vi "Data file Conversion.vi"() -> ()   [LabVIEW 2020]
uses:
  <vilib>/Utility/sysdir.llb/System Directory Type.ctl
  <vilib>/Utility/NIReport.llb/Report Type.ctl
  <vilib>/addons/_office/excel.llb/Excel Get Data ([str]).vi
  <vilib>/Utility/file.llb/Write Delimited Spreadsheet (string).vi
  <vilib>/Utility/NIReport.llb/NI_report.lvclass
  <vilib>/addons/_office/NI_ReportGenerationToolkit.lvlib
  <vilib>/Utility/NIReport.llb/Excel/NI_Excel.lvclass
  <vilib>/Utility/NIReport.llb/NI_ReportGenerationCore.lvlib
panel:
  out "data 2":string[][][](array[string])
  out "data":string[][](array[string])
  out "error out":errorcluster caption="에러 출력"
  in  "파일선택":T1(ring)=enum."Torque Weight Set"
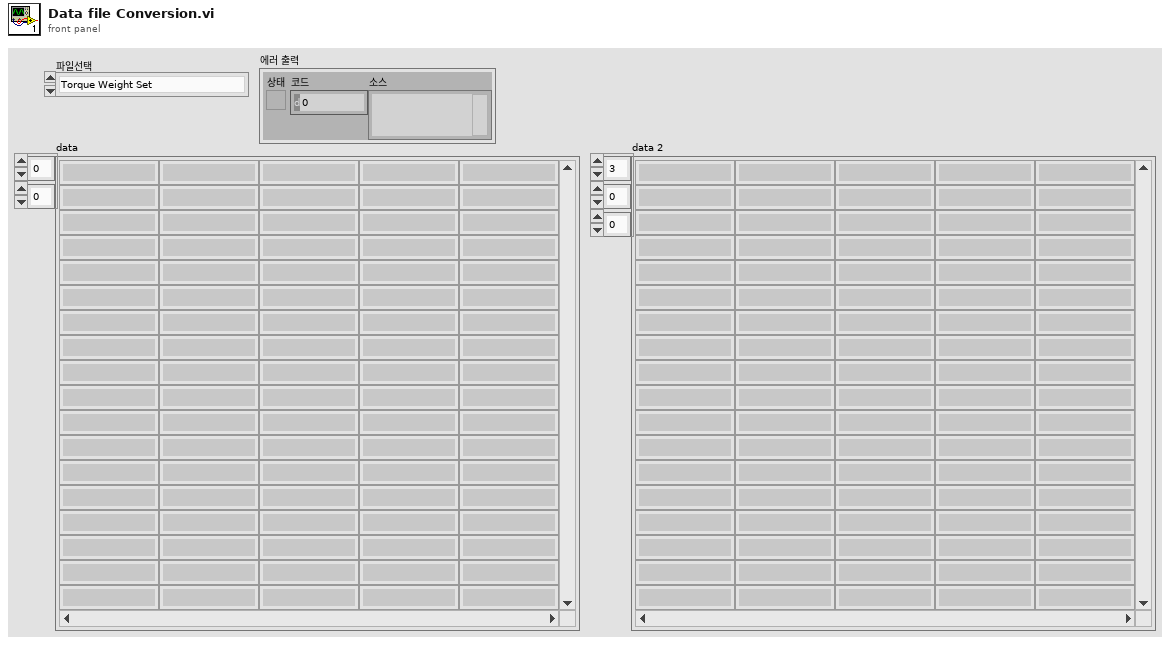
[diagram p1: front panel]
types:
  T1 = enum16{"Force Weight Set", "Torque Weight Set", "Deadweight Set", "Gauge Block Set", "Angle Gauge Block Set", "Thread Plug Gauge Set", "Surface Plate"}
  T2 = typedef "NI_ReportGenerationCore.lvlib/Report Type.ctl" = enum16{"HTML", "Word", "Excel"}
  T3 = enum16{"maximized", "minimized", "normal", "no change"}
  T4 = typedef "System Directory Type.ctl" = i32
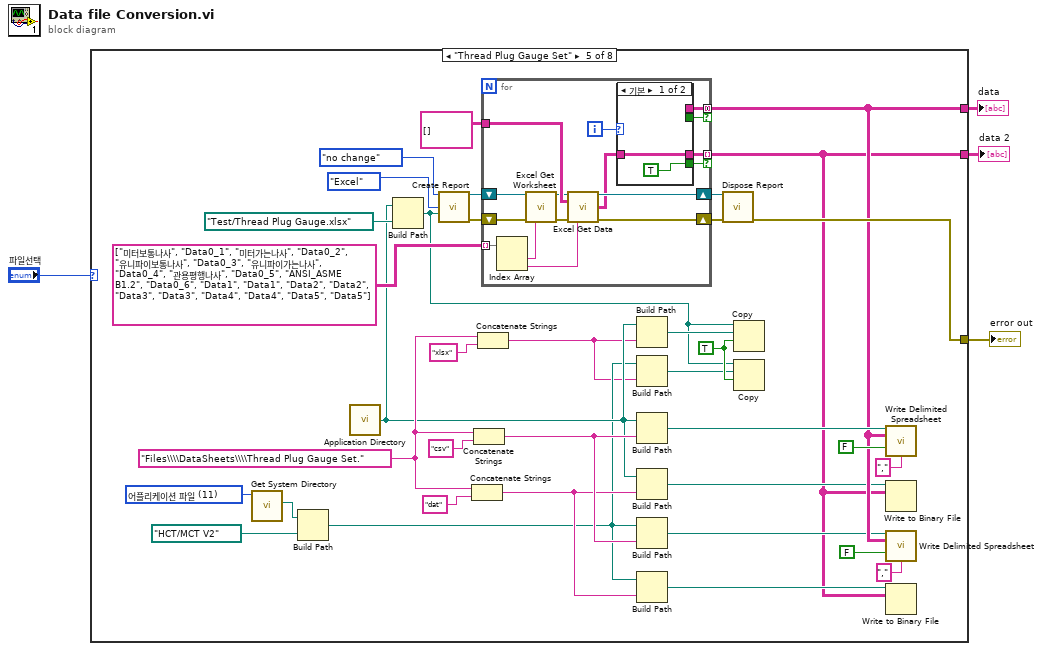
[diagram p0: block diagram]
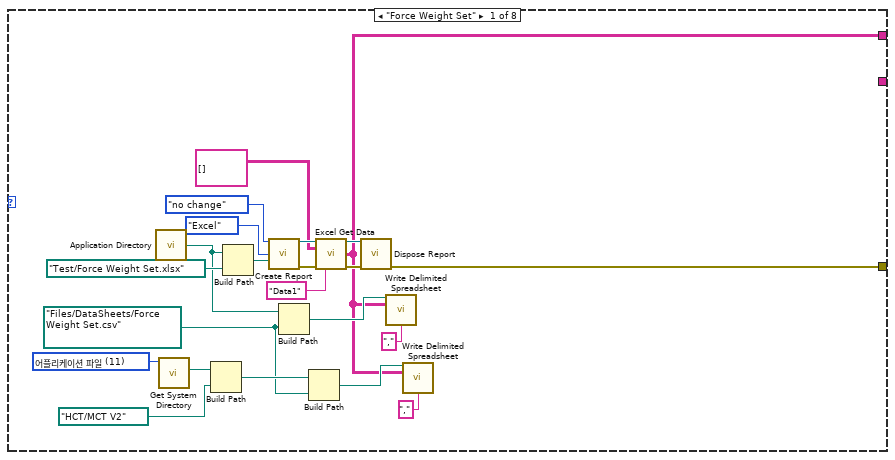
[diagram p2: hidden frame]
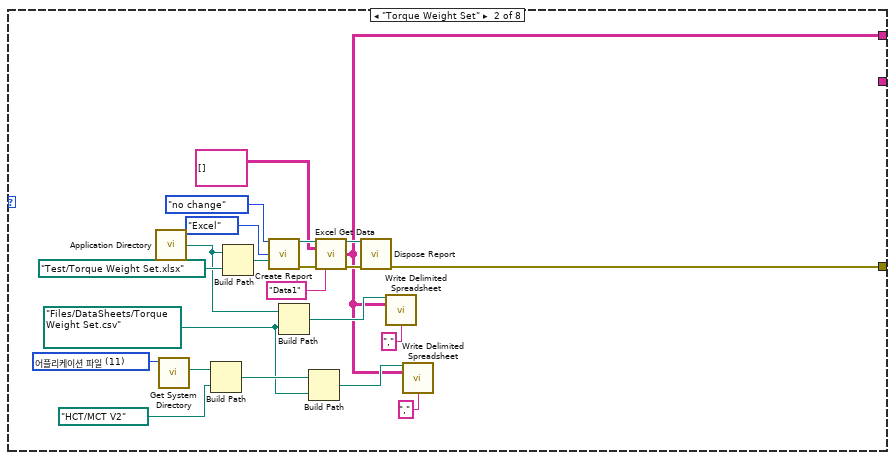
[diagram p3: hidden frame]
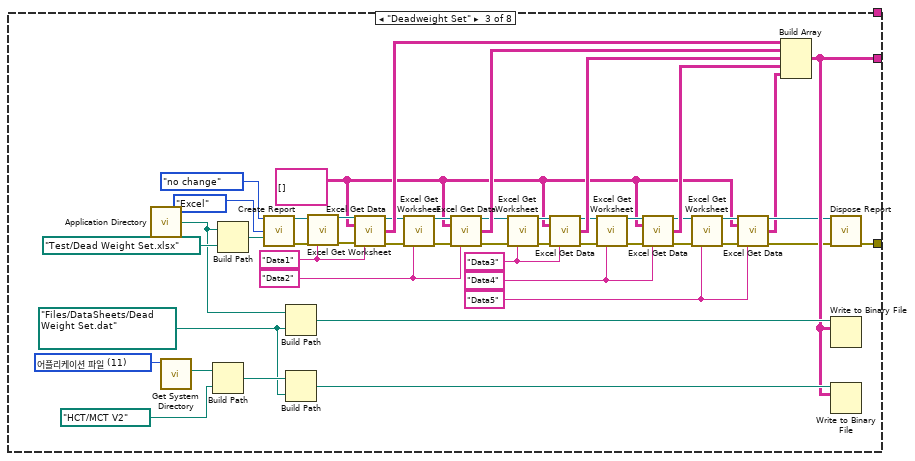
[diagram p4: hidden frame]
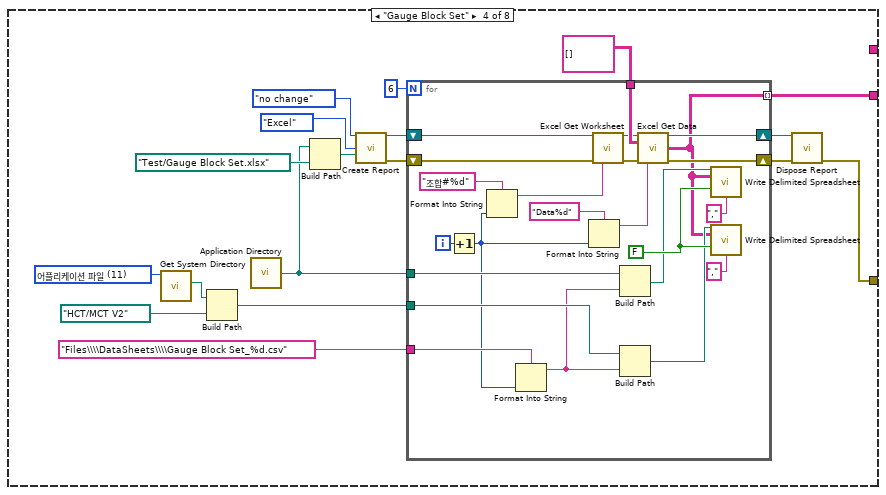
[diagram p5: hidden frame]
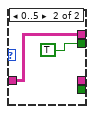
[diagram p6: hidden frame]
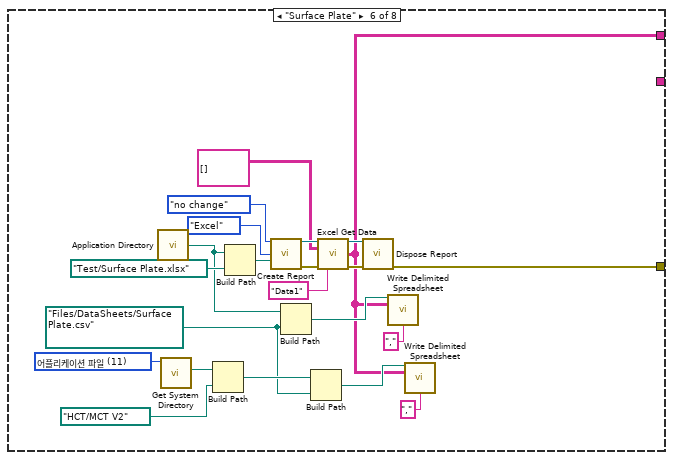
[diagram p7: hidden frame]
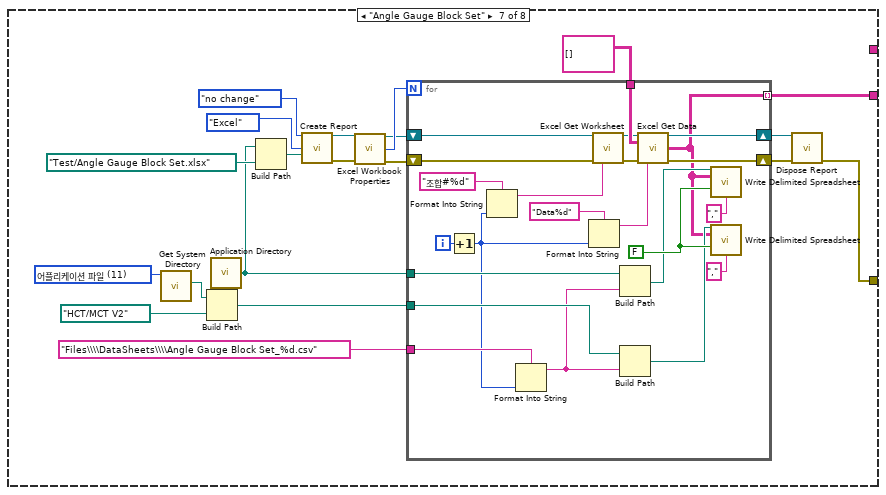
[diagram p8: hidden frame]
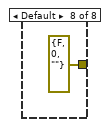
[diagram p9: hidden frame]
diagram:
  n1 = case shown="\"Thread Plug Gauge Set\"" "파일선택" {
    tunnel: [w14 w36 w91 w110 w170 w194 w231 errorcluster {"status"=FALSE, "code"=0, "source"=""} ("error out")] -> w3
    tunnel: [w6 w28 _ _ w151 w193 _ _] -> w2
    tunnel: [_ _ w65 w99 w147 _ w222 _] -> w1
    frame "Force Weight Set" {
      w13 = T4 11 items=["사용자 홈"=0, "사용자 데스크탑"=1, "사용자 문서"=2, "사용자 어플리케이션 데이터"=3, "사용자 환경"=4, "사용자 임시"=5, "퍼블릭 문서"=6, "퍼블릭 어플리케이션 데이터"=7, "퍼블릭 환경"=8, "퍼블릭 캐시"=13, "시스템 코어 라이브러리"=9, "시스템 설치된 라이브러리"=10, "어플리케이션 파일"=11, "부팅 볼륨 루트"=12] ("system directory type")
      w7 = path "Files/DataSheets/Force Weight Set.csv" ("경로")
      n2 = call <vilib>:"Application Directory.vi"() -> ("Application Directory"=w17:path)
      n3 = call <vilib>:"Get System Directory.vi"("system directory type"=w13) -> ("system directory"=w10:path)  [unwired: 10 in]
      n4 = Build Path(base path=w10, name or relative path=path "HCT/MCT V2" ("이름 또는 상대 경로")) -> (appended path=w8:path)
      n5 = Build Path(base path=w17, name or relative path=path "Test/Force Weight Set.xlsx" ("template (empty)")) -> (appended path=w24:path)
      n6 = call <vilib>:"Create Report.vi"("window state (normal)"=T3."no change", "report type"=Report_Type."Excel", "template (empty)"=w24) -> ("report out"=w22:refnum<class "NI_report.lvclass">, "error out"=w23:errorcluster)  [unwired: 11 in]
      n7 = Build Path(base path=w17, name or relative path=w7) -> (appended path=w16:path)
      n8 = Build Path(base path=w8, name or relative path=w7) -> (appended path=w11:path)
      n9 = call-poly <vilib>:"Excel Get Data.vi"("report in"=w22, "data type"=string[][] [], "error in (no error)"=w23, "name (\"\")"="Data1" ("machine name (empty)")) -> ("report out"=w20:refnum<class "NI_report.lvclass">, "data"=w6:string[][], "error out"=w19:errorcluster)  [unwired: 9 in]
      n10 = call-dynamic "Dispose Report.vi"("report in"=w20, "error in (no error)"=w19) -> ("error out"=w14:errorcluster)  [unwired: 13 in]
      n11 = call-poly <vilib>:"Write Delimited Spreadsheet.vi"("file path (dialog if empty)"=w16, "2D data"=w6, "delimiter (\\t)"="," ("delimiter (\\t)")) -> ()  [unwired: 11 in, 2 out]
      n12 = call-poly <vilib>:"Write Delimited Spreadsheet.vi"("file path (dialog if empty)"=w11, "2D data"=w6, "delimiter (\\t)"="," ("delimiter (\\t)")) -> ()  [unwired: 11 in, 2 out]
    }
    frame "Torque Weight Set" {
      w35 = T4 11 items=["사용자 홈"=0, "사용자 데스크탑"=1, "사용자 문서"=2, "사용자 어플리케이션 데이터"=3, "사용자 환경"=4, "사용자 임시"=5, "퍼블릭 문서"=6, "퍼블릭 어플리케이션 데이터"=7, "퍼블릭 환경"=8, "퍼블릭 캐시"=13, "시스템 코어 라이브러리"=9, "시스템 설치된 라이브러리"=10, "어플리케이션 파일"=11, "부팅 볼륨 루트"=12] ("system directory type")
      w29 = path "Files/DataSheets/Torque Weight Set.csv" ("경로")
      n13 = call <vilib>:"Application Directory.vi"() -> ("Application Directory"=w39:path)
      n14 = call <vilib>:"Get System Directory.vi"("system directory type"=w35) -> ("system directory"=w32:path)  [unwired: 10 in]
      n15 = Build Path(base path=w32, name or relative path=path "HCT/MCT V2" ("이름 또는 상대 경로")) -> (appended path=w30:path)
      n16 = Build Path(base path=w39, name or relative path=path "Test/Torque Weight Set.xlsx" ("template (empty)")) -> (appended path=w46:path)
      n17 = call <vilib>:"Create Report.vi"("window state (normal)"=T3."no change", "report type"=Report_Type."Excel", "template (empty)"=w46) -> ("report out"=w44:refnum<class "NI_report.lvclass">, "error out"=w45:errorcluster)  [unwired: 11 in]
      n18 = Build Path(base path=w39, name or relative path=w29) -> (appended path=w38:path)
      n19 = Build Path(base path=w30, name or relative path=w29) -> (appended path=w33:path)
      n20 = call-poly <vilib>:"Excel Get Data.vi"("report in"=w44, "data type"=string[][] [], "error in (no error)"=w45, "name (\"\")"="Data1" ("machine name (empty)")) -> ("report out"=w42:refnum<class "NI_report.lvclass">, "data"=w28:string[][], "error out"=w41:errorcluster)  [unwired: 9 in]
      n21 = call-dynamic "Dispose Report.vi"("report in"=w42, "error in (no error)"=w41) -> ("error out"=w36:errorcluster)  [unwired: 13 in]
      n22 = call-poly <vilib>:"Write Delimited Spreadsheet.vi"("file path (dialog if empty)"=w38, "2D data"=w28, "delimiter (\\t)"="," ("delimiter (\\t)")) -> ()  [unwired: 11 in, 2 out]
      n23 = call-poly <vilib>:"Write Delimited Spreadsheet.vi"("file path (dialog if empty)"=w33, "2D data"=w28, "delimiter (\\t)"="," ("delimiter (\\t)")) -> ()  [unwired: 11 in, 2 out]
    }
    frame "Deadweight Set" {
      w51 = "Data5" ("machine name (empty)")
      w59 = "Data4" ("machine name (empty)")
      w71 = T4 11 items=["사용자 홈"=0, "사용자 데스크탑"=1, "사용자 문서"=2, "사용자 어플리케이션 데이터"=3, "사용자 환경"=4, "사용자 임시"=5, "퍼블릭 문서"=6, "퍼블릭 어플리케이션 데이터"=7, "퍼블릭 환경"=8, "퍼블릭 캐시"=13, "시스템 코어 라이브러리"=9, "시스템 설치된 라이브러리"=10, "어플리케이션 파일"=11, "부팅 볼륨 루트"=12] ("system directory type")
      w72 = "Data3" ("machine name (empty)")
      w77 = "Data2" ("machine name (empty)")
      w67 = path "Files/DataSheets/Dead Weight Set.dat" ("경로")
      w50 = string[][] []
      w82 = "Data1" ("machine name (empty)")
      n24 = call <vilib>:"Application Directory.vi"() -> ("Application Directory"=w92:path)
      n25 = call <vilib>:"Get System Directory.vi"("system directory type"=w71) -> ("system directory"=w70:path)  [unwired: 10 in]
      n26 = Build Path(base path=w70, name or relative path=path "HCT/MCT V2" ("이름 또는 상대 경로")) -> (appended path=w68:path)
      n27 = Build Path(base path=w92, name or relative path=path "Test/Dead Weight Set.xlsx" ("template (empty)")) -> (appended path=w93:path)
      n28 = call <vilib>:"Create Report.vi"("window state (normal)"=T3."no change", "report type"=Report_Type."Excel", "template (empty)"=w93) -> ("report out"=w86:refnum<class "NI_report.lvclass">, "error out"=w85:errorcluster)  [unwired: 11 in]
      n29 = Build Path(base path=w92, name or relative path=w67) -> (appended path=w87:path)
      n30 = Build Path(base path=w68, name or relative path=w67) -> (appended path=w66:path)
      n31 = call <vilib>:"Excel Get Worksheet.vi"("report in"=w86, "error in (no error)"=w85, "name (\"\")"=w82) -> ("report out"=w83:refnum<class "NI_report.lvclass">, "error out"=w84:errorcluster)  [unwired: 11 in]
      n32 = call-poly <vilib>:"Excel Get Data.vi"("report in"=w83, "data type"=w50, "error in (no error)"=w84, "name (\"\")"=w82) -> ("report out"=w81:refnum<class "NI_report.lvclass">, "data"=w90:string[][], "error out"=w80:errorcluster)  [unwired: 9 in]
      n33 = call <vilib>:"Excel Get Worksheet.vi"("report in"=w81, "error in (no error)"=w80, "name (\"\")"=w77) -> ("report out"=w78:refnum<class "NI_report.lvclass">, "error out"=w79:errorcluster)  [unwired: 11 in]
      n34 = call-poly <vilib>:"Excel Get Data.vi"("report in"=w78, "data type"=w50, "error in (no error)"=w79, "name (\"\")"=w77) -> ("report out"=w76:refnum<class "NI_report.lvclass">, "data"=w89:string[][], "error out"=w75:errorcluster)  [unwired: 9 in]
      n35 = call <vilib>:"Excel Get Worksheet.vi"("report in"=w76, "error in (no error)"=w75, "name (\"\")"=w72) -> ("report out"=w74:refnum<class "NI_report.lvclass">, "error out"=w73:errorcluster)  [unwired: 11 in]
      n36 = call-poly <vilib>:"Excel Get Data.vi"("report in"=w74, "data type"=w50, "error in (no error)"=w73, "name (\"\")"=w72) -> ("report out"=w62:refnum<class "NI_report.lvclass">, "data"=w88:string[][], "error out"=w61:errorcluster)  [unwired: 9 in]
      n37 = call <vilib>:"Excel Get Worksheet.vi"("report in"=w62, "error in (no error)"=w61, "name (\"\")"=w59) -> ("report out"=w60:refnum<class "NI_report.lvclass">, "error out"=w63:errorcluster)  [unwired: 11 in]
      n38 = call-poly <vilib>:"Excel Get Data.vi"("report in"=w60, "data type"=w50, "error in (no error)"=w63, "name (\"\")"=w59) -> ("report out"=w56:refnum<class "NI_report.lvclass">, "data"=w58:string[][], "error out"=w55:errorcluster)  [unwired: 9 in]
      n39 = call <vilib>:"Excel Get Worksheet.vi"("report in"=w56, "error in (no error)"=w55, "name (\"\")"=w51) -> ("report out"=w54:refnum<class "NI_report.lvclass">, "error out"=w57:errorcluster)  [unwired: 11 in]
      n40 = call-poly <vilib>:"Excel Get Data.vi"("report in"=w54, "data type"=w50, "error in (no error)"=w57, "name (\"\")"=w51) -> ("report out"=w53:refnum<class "NI_report.lvclass">, "data"=w49:string[][], "error out"=w52:errorcluster)  [unwired: 9 in]
      n41 = Build Array(w90, w89, w88, w58, w49) -> (w65:string[][][])
      n42 = call-dynamic "Dispose Report.vi"("report in"=w53, "error in (no error)"=w52) -> ("error out"=w91:errorcluster)  [unwired: 13 in]
      n43 = Write to Binary File(file (use dialog)=w87, data=w65) -> ()  [unwired: 4 in, 3 out]
      n44 = Write to Binary File(file (use dialog)=w66, data=w65) -> ()  [unwired: 4 in, 3 out]
    }
    frame "Gauge Block Set" {
      w107 = T4 11 items=["사용자 홈"=0, "사용자 데스크탑"=1, "사용자 문서"=2, "사용자 어플리케이션 데이터"=3, "사용자 환경"=4, "사용자 임시"=5, "퍼블릭 문서"=6, "퍼블릭 어플리케이션 데이터"=7, "퍼블릭 환경"=8, "퍼블릭 캐시"=13, "시스템 코어 라이브러리"=9, "시스템 설치된 라이브러리"=10, "어플리케이션 파일"=11, "부팅 볼륨 루트"=12] ("system directory type")
      n45 = call <vilib>:"Get System Directory.vi"("system directory type"=w107) -> ("system directory"=w103:path)  [unwired: 10 in]
      n46 = Build Path(base path=w103, name or relative path=path "HCT/MCT V2" ("이름 또는 상대 경로")) -> (appended path=w101:path)
      n47 = call <vilib>:"Application Directory.vi"() -> ("Application Directory"=w100:path)
      n48 = Build Path(base path=w100, name or relative path=path "Test/Gauge Block Set.xlsx" ("template (empty)")) -> (appended path=w111:path)
      n49 = call <vilib>:"Create Report.vi"("window state (normal)"=T3."no change", "report type"=Report_Type."Excel", "template (empty)"=w111) -> ("report out"=w108:refnum<class "NI_report.lvclass">, "error out"=w109:errorcluster)  [unwired: 11 in]
      n50 = for {
        N: 6 -> [_]
        tunnel: string[][] [] -> [w132]
        shift-right: [w133] -> w105
        shift-left: w108 -> [w135]
        shift-right: [w136] -> w106
        shift-left: w109 -> [w134]
        tunnel: w101 -> [w125]
        tunnel: w100 -> [w123]
        tunnel: [w122] -> w99 mode=indexing
        tunnel: "Files\\\\DataSheets\\\\Gauge Block Set_%d.csv" -> [w116]
        i -> [w118]
        w127 = FALSE ("append to file? (new file:F)")
        n51 = Increment(x=w118) -> (x+1=w115:i32)
        n52 = Format Into String(format string="조합#%d", w115) -> (resulting string=w120:string)  [unwired: 2 in, 1 out]
        n53 = Format Into String(format string=w116, w115) -> (resulting string=w114:string)  [unwired: 2 in, 1 out]
        n54 = Format Into String(format string="Data%d", w115) -> (resulting string=w117:string)  [unwired: 2 in, 1 out]
        n55 = call <vilib>:"Excel Get Worksheet.vi"("report in"=w135, "error in (no error)"=w134, "name (\"\")"=w120) -> ("report out"=w129:refnum<class "NI_report.lvclass">, "error out"=w128:errorcluster)  [unwired: 11 in]
        n56 = Build Path(base path=w123, name or relative path=w114) -> (appended path=w124:path)
        n57 = Build Path(base path=w125, name or relative path=w114) -> (appended path=w126:path)
        n58 = call-poly <vilib>:"Excel Get Data.vi"("report in"=w129, "data type"=w132, "error in (no error)"=w128, "name (\"\")"=w117) -> ("report out"=w133:refnum<class "NI_report.lvclass">, "data"=w122:string[][], "error out"=w136:errorcluster)  [unwired: 9 in]
        n59 = call-poly <vilib>:"Write Delimited Spreadsheet.vi"("file path (dialog if empty)"=w124, "2D data"=w122, "append to file? (new file:F)"=w127, "delimiter (\\t)"="," ("delimiter (\\t)")) -> ()  [unwired: 10 in, 2 out]
        n60 = call-poly <vilib>:"Write Delimited Spreadsheet.vi"("file path (dialog if empty)"=w126, "2D data"=w122, "append to file? (new file:F)"=w127, "delimiter (\\t)"="," ("delimiter (\\t)")) -> ()  [unwired: 10 in, 2 out]
      }
      n61 = call-dynamic "Dispose Report.vi"("report in"=w105, "error in (no error)"=w106) -> ("error out"=w110:errorcluster)  [unwired: 13 in]
    }
    frame "Thread Plug Gauge Set" {
      w139 = TRUE ("덮어쓰기(거짓)")
      w144 = "Files\\\\DataSheets\\\\Thread Plug Gauge Set."
      w167 = T4 11 items=["사용자 홈"=0, "사용자 데스크탑"=1, "사용자 문서"=2, "사용자 어플리케이션 데이터"=3, "사용자 환경"=4, "사용자 임시"=5, "퍼블릭 문서"=6, "퍼블릭 어플리케이션 데이터"=7, "퍼블릭 환경"=8, "퍼블릭 캐시"=13, "시스템 코어 라이브러리"=9, "시스템 설치된 라이브러리"=10, "어플리케이션 파일"=11, "부팅 볼륨 루트"=12] ("system directory type")
      n62 = call <vilib>:"Get System Directory.vi"("system directory type"=w167) -> ("system directory"=w163:path)  [unwired: 10 in]
      n63 = Build Path(base path=w163, name or relative path=path "HCT/MCT V2" ("이름 또는 상대 경로")) -> (appended path=w141:path)
      n64 = call <vilib>:"Application Directory.vi"() -> ("Application Directory"=w143:path)
      n65 = Build Path(base path=w143, name or relative path=path "Test/Thread Plug Gauge.xlsx" ("template (empty)")) -> (appended path=w137:path)
      n66 = call <vilib>:"Create Report.vi"("window state (normal)"=T3."no change", "report type"=Report_Type."Excel", "template (empty)"=w137) -> ("report out"=w168:refnum<class "NI_report.lvclass">, "error out"=w169:errorcluster)  [unwired: 11 in]
      n67 = Concatenate Strings(w144, "dat" ("문자열")) -> (w146:string)
      n68 = Concatenate Strings(w144, "csv" ("문자열")) -> (w150:string)
      n69 = Concatenate Strings(w144, "xlsx" ("문자열")) -> (w140:string)
      n70 = for {
        tunnel: string[][] [] -> [w184]
        shift-right: [w185] -> w165
        shift-left: w168 -> [w187]
        shift-right: [w188] -> w166
        shift-left: w169 -> [w186]
        tunnel: [w175] -> w147 mode=indexing if=w173
        tunnel: string[][] [["미터보통나사", "Data0_1"], ["미터가는나사", "Data0_2"], ["유니파이보통나사", "Data0_3"], ["유니파이가는나사", "Data0_4"], ["관용평행나사", "Data0_5"], ["ANSI_ASME B1.2", "Data0_6"], ["Data1", "Data1"], ["Data2", "Data2"], ["Data3", "Data3"], ["Data4", "Data4"], ["Data5", "Data5"]] -> [w181] mode=indexing
        tunnel: [w176] -> w151 mode=concatenating if=w174
        i -> [w178]
        n71 = Index Array(array=w181) -> (element #1=w180:string, element #2=w179:string)  [unwired: 2 in]
        n72 = call <vilib>:"Excel Get Worksheet.vi"("report in"=w187, "error in (no error)"=w186, "name (\"\")"=w180) -> ("report out"=w183:refnum<class "NI_report.lvclass">, "error out"=w182:errorcluster)  [unwired: 11 in]
        n73 = call-poly <vilib>:"Excel Get Data.vi"("report in"=w183, "data type"=w184, "error in (no error)"=w182, "name (\"\")"=w179) -> ("report out"=w185:refnum<class "NI_report.lvclass">, "data"=w177:string[][], "error out"=w188:errorcluster)  [unwired: 9 in]
        n74 = case shown="기본" w178 {
          tunnel: w177 -> [w190 w192]
          tunnel: [_ w192] -> w176
          tunnel: [w190 _] -> w175
          tunnel: [_ TRUE] -> w174
          tunnel: [TRUE _] -> w173
          frame Default {
          }
          frame 0..5 {
          }
        }
      }
      n75 = Build Path(base path=w143, name or relative path=w140) -> (appended path=w142:path)
      n76 = Build Path(base path=w141, name or relative path=w140) -> (appended path=w138:path)
      n77 = Build Path(base path=w143, name or relative path=w150) -> (appended path=w159:path)
      n78 = Build Path(base path=w143, name or relative path=w146) -> (appended path=w148:path)
      n79 = Build Path(base path=w141, name or relative path=w150) -> (appended path=w149:path)
      n80 = Build Path(base path=w141, name or relative path=w146) -> (appended path=w157:path)
      n81 = call-dynamic "Dispose Report.vi"("report in"=w165, "error in (no error)"=w166) -> ("error out"=w170:errorcluster)  [unwired: 13 in]
      n82 = Copy(9:w139, 10:w142, 11:w137) -> ()  [unwired: 2 in, 3 out]
      n83 = Copy(9:w139, 10:w138, 11:w137) -> ()  [unwired: 2 in, 3 out]
      n84 = call-poly <vilib>:"Write Delimited Spreadsheet.vi"("file path (dialog if empty)"=w159, "2D data"=w151, "append to file? (new file:F)"=FALSE, "delimiter (\\t)"="," ("delimiter (\\t)")) -> ()  [unwired: 10 in, 2 out]
      n85 = Write to Binary File(file (use dialog)=w148, data=w147) -> ()  [unwired: 4 in, 3 out]
      n86 = call-poly <vilib>:"Write Delimited Spreadsheet.vi"("file path (dialog if empty)"=w149, "2D data"=w151, "append to file? (new file:F)"=FALSE, "delimiter (\\t)"="," ("delimiter (\\t)")) -> ()  [unwired: 10 in, 2 out]
      n87 = Write to Binary File(file (use dialog)=w157, data=w147) -> ()  [unwired: 4 in, 3 out]
    }
    frame "Surface Plate" {
      w202 = T4 11 items=["사용자 홈"=0, "사용자 데스크탑"=1, "사용자 문서"=2, "사용자 어플리케이션 데이터"=3, "사용자 환경"=4, "사용자 임시"=5, "퍼블릭 문서"=6, "퍼블릭 어플리케이션 데이터"=7, "퍼블릭 환경"=8, "퍼블릭 캐시"=13, "시스템 코어 라이브러리"=9, "시스템 설치된 라이브러리"=10, "어플리케이션 파일"=11, "부팅 볼륨 루트"=12] ("system directory type")
      w196 = path "Files/DataSheets/Surface Plate.csv" ("경로")
      n88 = call <vilib>:"Application Directory.vi"() -> ("Application Directory"=w205:path)
      n89 = call <vilib>:"Get System Directory.vi"("system directory type"=w202) -> ("system directory"=w199:path)  [unwired: 10 in]
      n90 = Build Path(base path=w199, name or relative path=path "HCT/MCT V2" ("이름 또는 상대 경로")) -> (appended path=w197:path)
      n91 = Build Path(base path=w205, name or relative path=path "Test/Surface Plate.xlsx" ("template (empty)")) -> (appended path=w212:path)
      n92 = call <vilib>:"Create Report.vi"("window state (normal)"=T3."no change", "report type"=Report_Type."Excel", "template (empty)"=w212) -> ("report out"=w210:refnum<class "NI_report.lvclass">, "error out"=w211:errorcluster)  [unwired: 11 in]
      n93 = Build Path(base path=w205, name or relative path=w196) -> (appended path=w204:path)
      n94 = Build Path(base path=w197, name or relative path=w196) -> (appended path=w200:path)
      n95 = call-poly <vilib>:"Excel Get Data.vi"("report in"=w210, "data type"=string[][] [], "error in (no error)"=w211, "name (\"\")"="Data1" ("machine name (empty)")) -> ("report out"=w208:refnum<class "NI_report.lvclass">, "data"=w193:string[][], "error out"=w207:errorcluster)  [unwired: 9 in]
      n96 = call-dynamic "Dispose Report.vi"("report in"=w208, "error in (no error)"=w207) -> ("error out"=w194:errorcluster)  [unwired: 13 in]
      n97 = call-poly <vilib>:"Write Delimited Spreadsheet.vi"("file path (dialog if empty)"=w204, "2D data"=w193, "delimiter (\\t)"="," ("delimiter (\\t)")) -> ()  [unwired: 11 in, 2 out]
      n98 = call-poly <vilib>:"Write Delimited Spreadsheet.vi"("file path (dialog if empty)"=w200, "2D data"=w193, "delimiter (\\t)"="," ("delimiter (\\t)")) -> ()  [unwired: 11 in, 2 out]
    }
    frame "Angle Gauge Block Set" {
      w230 = T4 11 items=["사용자 홈"=0, "사용자 데스크탑"=1, "사용자 문서"=2, "사용자 어플리케이션 데이터"=3, "사용자 환경"=4, "사용자 임시"=5, "퍼블릭 문서"=6, "퍼블릭 어플리케이션 데이터"=7, "퍼블릭 환경"=8, "퍼블릭 캐시"=13, "시스템 코어 라이브러리"=9, "시스템 설치된 라이브러리"=10, "어플리케이션 파일"=11, "부팅 볼륨 루트"=12] ("system directory type")
      n99 = call <vilib>:"Get System Directory.vi"("system directory type"=w230) -> ("system directory"=w226:path)  [unwired: 10 in]
      n100 = Build Path(base path=w226, name or relative path=path "HCT/MCT V2" ("이름 또는 상대 경로")) -> (appended path=w224:path)
      n101 = call <vilib>:"Application Directory.vi"() -> ("Application Directory"=w223:path)
      n102 = Build Path(base path=w223, name or relative path=path "Test/Angle Gauge Block Set.xlsx" ("template (empty)")) -> (appended path=w232:path)
      n103 = call <vilib>:"Create Report.vi"("window state (normal)"=T3."no change", "report type"=Report_Type."Excel", "template (empty)"=w232) -> ("report out"=w219:refnum<class "NI_report.lvclass">, "error out"=w218:errorcluster)  [unwired: 11 in]
      n104 = call <vilib>:"Excel Workbook Properties.vi"("report in"=w219, "error in (no error)"=w218) -> ("report out"=w216:refnum<class "NI_report.lvclass">, "worksheets count"=w217:i32, "error out"=w215:errorcluster)  [unwired: 10 in, 1 out]
      n105 = for {
        N: w217 -> [_]
        tunnel: string[][] [] -> [w253]
        shift-right: [w254] -> w228
        shift-left: w216 -> [w256]
        shift-right: [w257] -> w229
        shift-left: w215 -> [w255]
        tunnel: w224 -> [w246]
        tunnel: w223 -> [w244]
        tunnel: [w243] -> w222 mode=indexing
        tunnel: "Files\\\\DataSheets\\\\Angle Gauge Block Set_%d.csv" -> [w237]
        i -> [w239]
        w248 = FALSE ("append to file? (new file:F)")
        n106 = Increment(x=w239) -> (x+1=w236:i32)
        n107 = Format Into String(format string="조합#%d", w236) -> (resulting string=w241:string)  [unwired: 2 in, 1 out]
        n108 = Format Into String(format string=w237, w236) -> (resulting string=w235:string)  [unwired: 2 in, 1 out]
        n109 = Format Into String(format string="Data%d", w236) -> (resulting string=w238:string)  [unwired: 2 in, 1 out]
        n110 = call <vilib>:"Excel Get Worksheet.vi"("report in"=w256, "error in (no error)"=w255, "name (\"\")"=w241) -> ("report out"=w250:refnum<class "NI_report.lvclass">, "error out"=w249:errorcluster)  [unwired: 11 in]
        n111 = Build Path(base path=w244, name or relative path=w235) -> (appended path=w245:path)
        n112 = Build Path(base path=w246, name or relative path=w235) -> (appended path=w247:path)
        n113 = call-poly <vilib>:"Excel Get Data.vi"("report in"=w250, "data type"=w253, "error in (no error)"=w249, "name (\"\")"=w238) -> ("report out"=w254:refnum<class "NI_report.lvclass">, "data"=w243:string[][], "error out"=w257:errorcluster)  [unwired: 9 in]
        n114 = call-poly <vilib>:"Write Delimited Spreadsheet.vi"("file path (dialog if empty)"=w245, "2D data"=w243, "append to file? (new file:F)"=w248, "delimiter (\\t)"="," ("delimiter (\\t)")) -> ()  [unwired: 10 in, 2 out]
        n115 = call-poly <vilib>:"Write Delimited Spreadsheet.vi"("file path (dialog if empty)"=w247, "2D data"=w243, "append to file? (new file:F)"=w248, "delimiter (\\t)"="," ("delimiter (\\t)")) -> ()  [unwired: 10 in, 2 out]
      }
      n116 = call-dynamic "Dispose Report.vi"("report in"=w228, "error in (no error)"=w229) -> ("error out"=w231:errorcluster)  [unwired: 13 in]
    }
    frame Default {
    }
  }
  "error out" <- w3
  "data" <- w2
  "data 2" <- w1
